vi "Flatten Message To String.vi"(0 "message":T1, 11 "error in":errorcluster) -> (4 "message string":string, 15 "error out":errorcluster)   [LabVIEW 2009, in "AMC.lvlib"]
uses:
  AMC.lvlib
  Message.ctl
  <vilib>/NI/Tools/Keyed Array/KeyedArray.ctl
  <vilib>/NI/Tools/Keyed Array/Tools_KeyedArray.lvlib
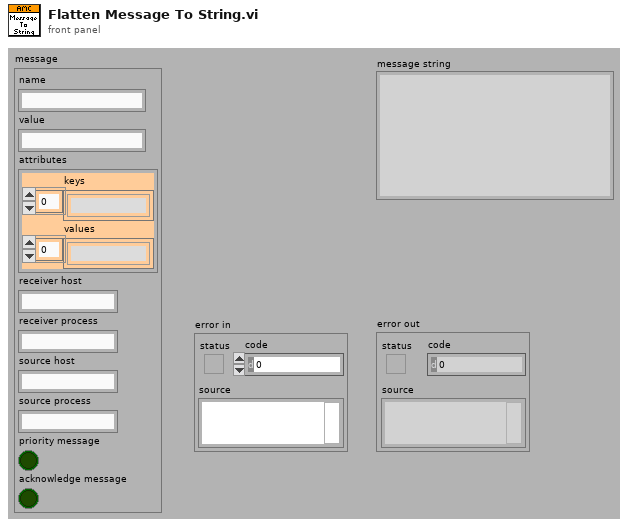
[diagram p1: front panel]
types:
  T1 = typedef "AMC.lvlib/Message.ctl" = cluster{"name":string, "value":string, "attributes":T2, "receiver host":string, "receiver process":string, "source host":string, "source process":string, "priority message":bool, "acknowledge message":bool}
  T2 = typedef "Tools_KeyedArray.lvlib/KeyedArray.ctl" = cluster{"keys":string[], "values":string[]}
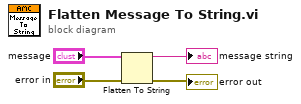
[diagram p0: block diagram]
diagram:
  n1 = Flatten To String(anything="message", error in (no error)="error in") -> (data string=→"message string":string, error out=→"error out":errorcluster)  [unwired: 2 in, 1 out]
